vi "ReadObjectLayout.vi"(7 "properties to ignore":variant, 8 "error in (no error)":errorcluster, 10 "GObj Refnum":refnum<vi>, 11 "Control Layout in":refnum<class "Listbox Control Layout.lvclass">) -> (0 "error out":errorcluster, 3 "Control Layout out":refnum<class "Listbox Control Layout.lvclass">)   [LabVIEW 2010, in "NI_SE_Front Panel Layout.lvlib" / "Listbox Control Layout.lvclass"]
doc: "Read layout information from the GObj Refnum."
uses:
  Listbox Control Layout.lvclass
  Control Layout/Control Layout.lvclass
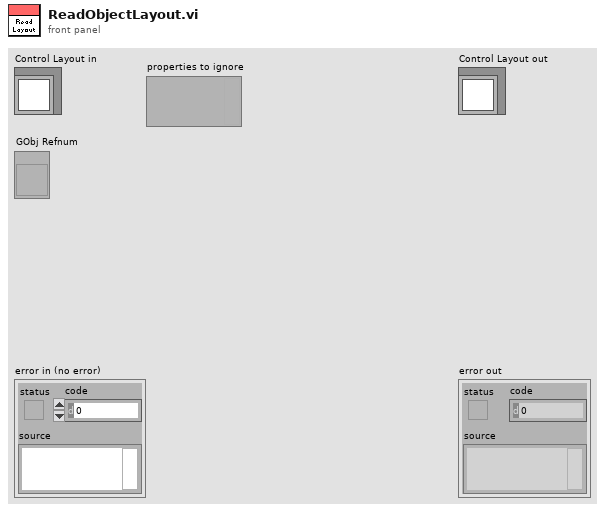
[diagram p1: front panel]
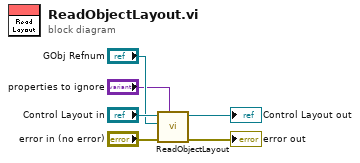
[diagram p0: block diagram]
diagram:
  n1 = call-parent "ReadObjectLayout.vi"("properties to ignore"="properties to ignore", "error in (no error)"="error in (no error)", "GObj Refnum"="GObj Refnum", "Control Layout in"="Control Layout in") -> ("error out"=→"error out":errorcluster, "Control Layout out"=→"Control Layout out":refnum<class "Listbox Control Layout.lvclass">)  [unwired: 6 in]
